vi "Set Action.vi"(8 "error in (no error)":errorcluster, 10 "Action":refnum<class "Action.lvclass">, 11 "Message in":refnum<class "Message.lvclass">) -> (0 "error out":errorcluster, 3 "Message out":refnum<class "Message.lvclass">)   [LabVIEW 2018, in "Message.lvclass"]
uses:
  Message.lvclass
  Action_class/Action.lvclass
  Message.lvclass/Message.ctl
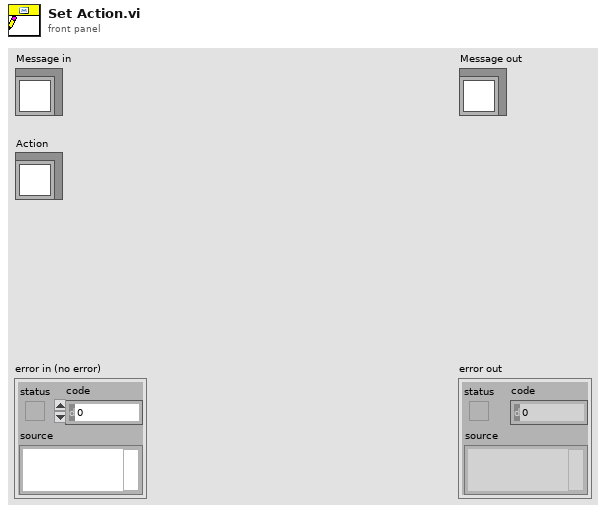
[diagram p1: front panel]
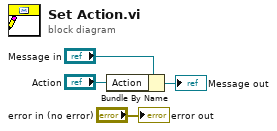
[diagram p0: block diagram]
diagram:
  n1 = Bundle By Name(cluster="Message in", "Action"="Action") -> (→"Message out":refnum<class "Message.lvclass">)
  "error out" <- "error in (no error)"
